vi "TX_Logic.vi"(6 "initialized array 2":dbl[](array[numeric]), 9 "VISA resource name":refnum<visa-resource-name>) -> (3 "read buffer":string)   [LabVIEW 2024]
uses:
  <vilib>/Instr/_visa.llb/VISA Configure Serial Port (Instr).vi
panel:
  out "error out 2":errorcluster
  out "Boolean":bool
  out "error out":errorcluster
  out "return count":u32
  out "String":string
  in  "baud rate (9600)":u32=9600
  out "result":dbl
  out "element 11":dbl
  out "element 10":dbl
  out "element 9":dbl
  out "element 8":dbl
  out "element 7":dbl
  out "element 6":dbl
  out "element 5":dbl
  out "element 4":dbl
  out "element 3":dbl
  out "element 2":dbl
  out "element":dbl
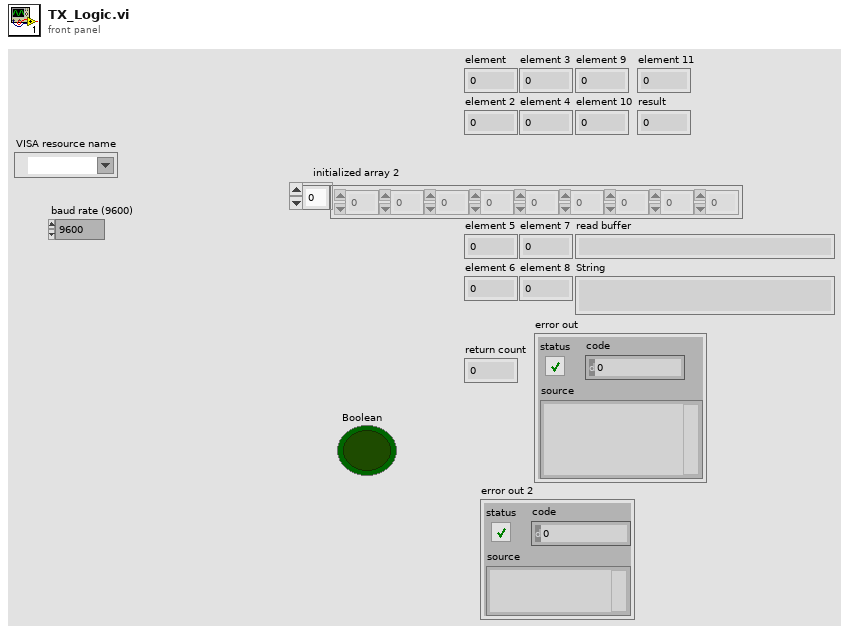
[diagram p1: front panel]
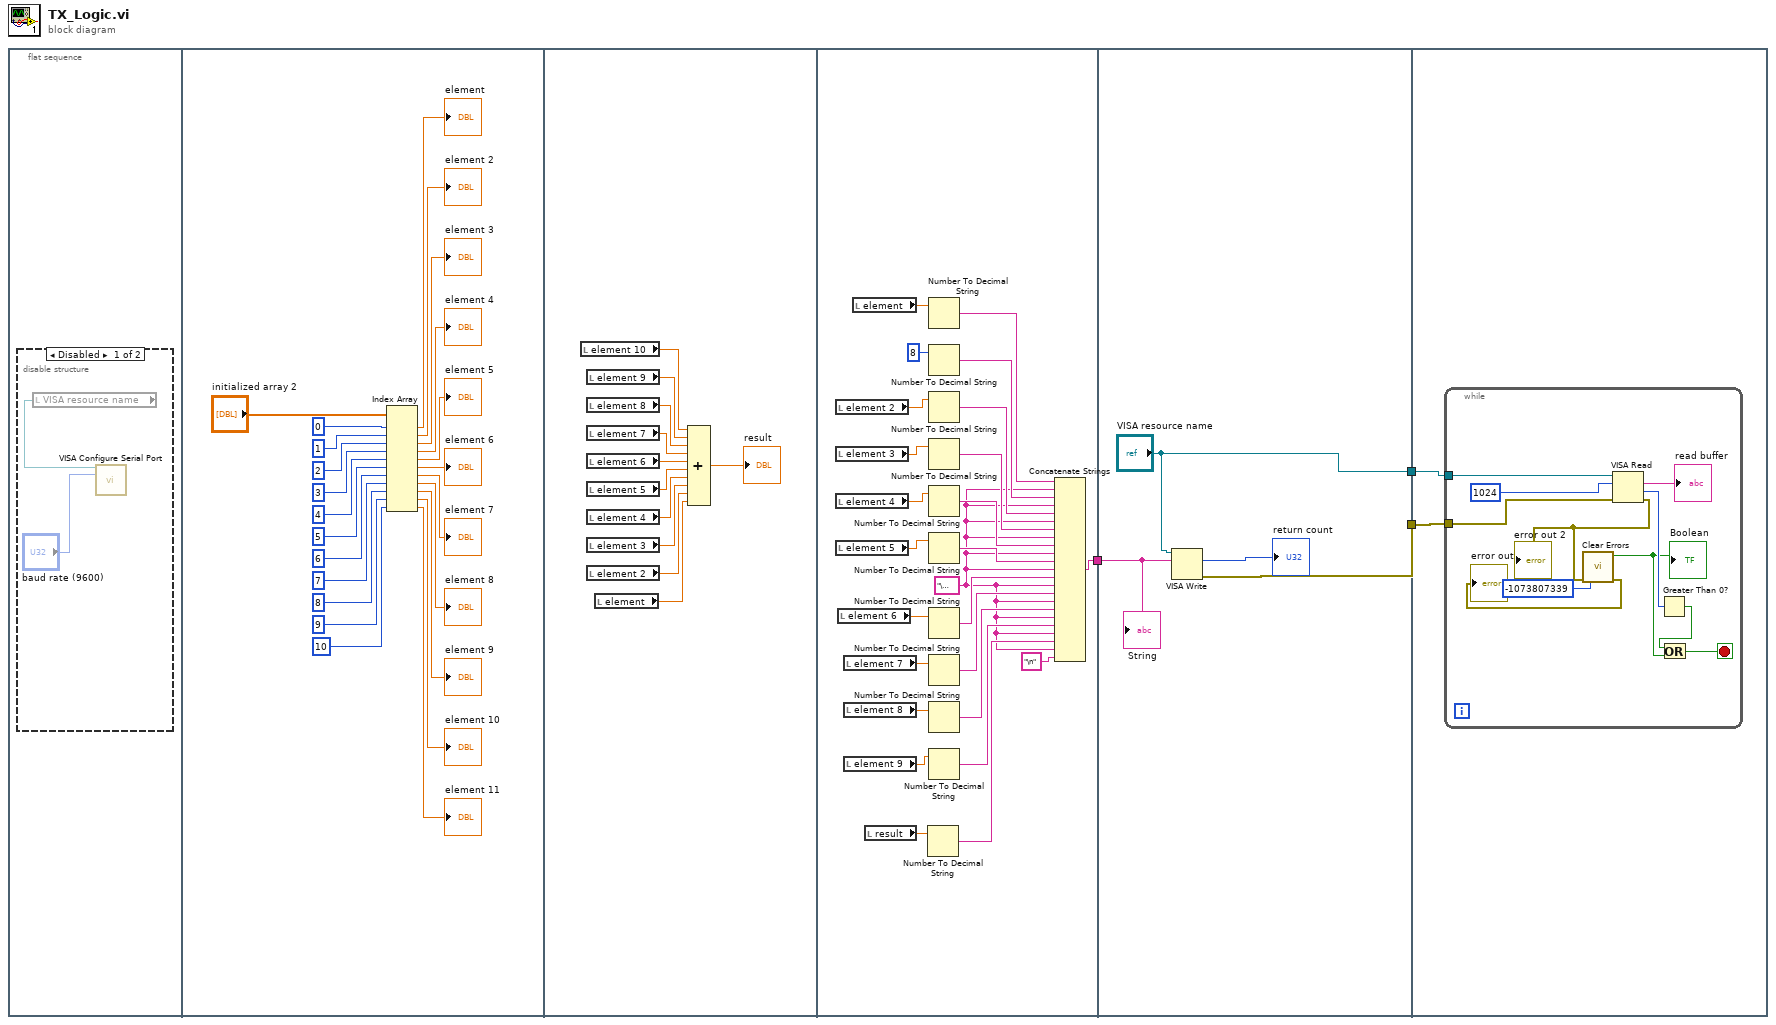
[diagram p0: block diagram]
diagram:
  n1 = flat-sequence {
    tunnel: [w53] -> w3
    tunnel: w3 -> [w68]
    tunnel: ["VISA resource name"] -> w2
    tunnel: [w66] -> w1
    tunnel: w2 -> [w70]
    tunnel: w1 -> [w69]
    frame #0 {
      n2 = disable-structure shown="Disabled" {
        frame Disabled {
          n3 = local read "VISA resource name"() -> (w5:refnum<visa-resource-name>)
          n4 = call-poly "VISA Configure Serial Port"("VISA resource name"=w5, "baud rate (9600)"="baud rate (9600)") -> ()  [unwired: 12 in, 2 out]
        }
        frame Enabled {
        }
      }
    }
    frame #1 {
      n5 = Index Array(array="initialized array 2", index #1=0 ("index"), index #2=1 ("index"), index #3=2 ("index"), index #4=3 ("index"), index #5=4 ("index"), index #6=5 ("index"), index #7=6 ("index"), index #8=7 ("index"), index #9=8 ("index"), index #10=9 ("index"), index #11=10 ("index")) -> (element #1=→"element":dbl, element #2=→"element 2":dbl, element #3=→"element 3":dbl, element #4=→"element 4":dbl, element #5=→"element 5":dbl, element #6=→"element 6":dbl, element #7=→"element 7":dbl, element #8=→"element 8":dbl, element #9=→"element 9":dbl, element #10=→"element 10":dbl, element #11=→"element 11":dbl)
    }
    frame #2 {
      n6 = local read "element 10"() -> (w30:dbl)
      n7 = local read "element 9"() -> (w31:dbl)
      n8 = local read "element 8"() -> (w32:dbl)
      n9 = local read "element 7"() -> (w33:dbl)
      n10 = local read "element 6"() -> (w34:dbl)
      n11 = local read "element 5"() -> (w35:dbl)
      n12 = local read "element 4"() -> (w36:dbl)
      n13 = local read "element 3"() -> (w37:dbl)
      n14 = local read "element 2"() -> (w38:dbl)
      n15 = local read "element"() -> (w39:dbl)
      n16 = Compound Arithmetic op=ADD(w30, w31, w32, w33, w34, w35, w36, w37, w38, w39) -> (→"result":dbl)
    }
    frame #3 {
      w50 = "\u0000"
      n17 = local read "element 2"() -> (w41:dbl)
      n18 = local read "element 3"() -> (w42:dbl)
      n19 = local read "element 4"() -> (w43:dbl)
      n20 = local read "element 5"() -> (w44:dbl)
      n21 = local read "element 6"() -> (w45:dbl)
      n22 = local read "element 7"() -> (w46:dbl)
      n23 = local read "element 8"() -> (w47:dbl)
      n24 = local read "element 9"() -> (w48:dbl)
      n25 = local read "element"() -> (w64:dbl)
      n26 = local read "result"() -> (w52:dbl)
      n27 = Number To Decimal String(number=w52) -> (decimal integer string=w51:string)  [unwired: 1 in]
      n28 = Number To Decimal String(number=w64) -> (decimal integer string=w63:string)  [unwired: 1 in]
      n29 = Number To Decimal String(number=8) -> (decimal integer string=w62:string)  [unwired: 1 in]
      n30 = Number To Decimal String(number=w41) -> (decimal integer string=w61:string)  [unwired: 1 in]
      n31 = Number To Decimal String(number=w42) -> (decimal integer string=w60:string)  [unwired: 1 in]
      n32 = Number To Decimal String(number=w43) -> (decimal integer string=w59:string)  [unwired: 1 in]
      n33 = Number To Decimal String(number=w44) -> (decimal integer string=w58:string)  [unwired: 1 in]
      n34 = Number To Decimal String(number=w45) -> (decimal integer string=w57:string)  [unwired: 1 in]
      n35 = Number To Decimal String(number=w46) -> (decimal integer string=w56:string)  [unwired: 1 in]
      n36 = Number To Decimal String(number=w47) -> (decimal integer string=w55:string)  [unwired: 1 in]
      n37 = Number To Decimal String(number=w48) -> (decimal integer string=w54:string)  [unwired: 1 in]
      n38 = Concatenate Strings(w63, w50, w62, w50, w61, w50, w60, w50, w59, w50, w58, w50, w57, w50, w56, w50, w55, w50, w54, w50, w51, w50, "\n") -> (w53:string)
    }
    frame #4 {
      n39 = VISA Write(VISA resource name="VISA resource name", write buffer=w68) -> (return count=→"return count":u32, error out=w66:errorcluster)  [unwired: 1 in, 1 out]
      "String" <- w68
    }
    frame #5 {
      n40 = while {
        tunnel: w70 -> [w77]
        tunnel: w69 -> [w78]
        stop <- w71 stop-if-true
        n41 = VISA Read(VISA resource name=w77, byte count=u32 1024, error in (no error)=w78) -> (read buffer=→"read buffer":string, return count=w79:u32, error out=w76:errorcluster)  [unwired: 1 out]
        "error out 2" <- w76
        n42 = call <vilib>:"Clear Errors.vi"("error in (no error)"=w76, "specific error code to clear (0: all)"=-1073807339) -> ("error out"=→"error out":errorcluster, "specific error cleared?"=w72:bool)  [unwired: 4 in]
        "Boolean" <- w72
        n43 = Greater Than 0?(x=w79) -> (x > 0?=w73:bool)
        n44 = Or(x=w73, y=w72) -> (x .or. y?=w71:bool)
      }
    }
  }
